vi "Configure Session.vi"(8 "error in":errorcluster, 11 "Plugin in":refnum<class "StreamWriter.lvclass">) -> (0 "error out":errorcluster, 3 "Plugin out":refnum<class "StreamWriter.lvclass">)   [LabVIEW 2024, in "StreamWriter.lvlib" / "StreamWriter.lvclass"]
uses:
  StreamWriter.lvclass
  C:/Program Files/National Instruments/LabVIEW 2024/vi.lib/FlexLogger/SDK/PluginSDK.lvlibp/PEFClasses/SDK/Plugin/Plugin.lvclass
  StreamWriter Parameters.ctl
  StreamWriter.lvclass/StreamWriter.ctl
  StreamWriter Strings.vi
  <vilib>/FlexLogger/SDK/PluginSDK.lvlibp/PEFClasses/SDK/Plugin/ParameterAccess/Read I32.vi
  <vilib>/FlexLogger/SDK/PluginSDK.lvlibp/PEFClasses/SDK/Plugin/Plugin.lvclass
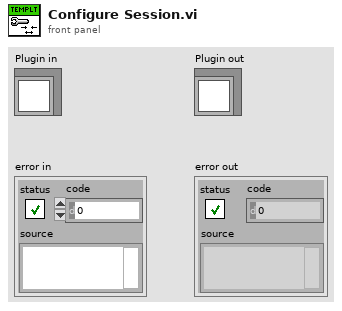
[diagram p1: front panel]
types:
  T1 = typedef "StreamWriter.lvlib/StreamWriter.lvclass/StreamWriter Parameters.ctl" = cluster{"Timeout":i32, "Buffer Size":i32, "Writer Endpoint":refnum<k21>}
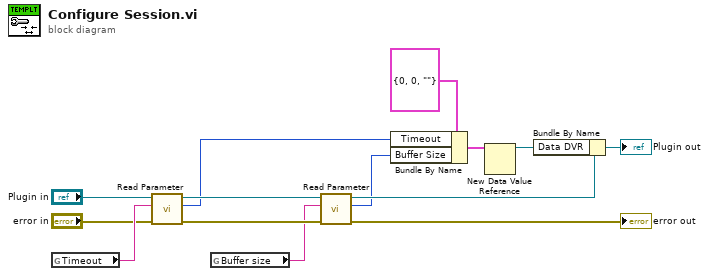
[diagram p0: block diagram]
diagram:
  n1 = global read "StreamWriter Strings.vi" "Timeout"() -> (w5:string)
  n2 = call-poly <vilib>:"Read Parameter.vi"("error in (no error)"="error in", "Name"=w5, "Plugin in"="Plugin in") -> ("error out"=w13:errorcluster, "Value"=w11:i32, "Plugin out"=w14:refnum<class "StreamWriter.lvclass">)  [unwired: 5 in, 1 out]
  n3 = global read "StreamWriter Strings.vi" "Buffer size"() -> (w4:string)
  n4 = call-poly <vilib>:"Read Parameter.vi"("error in (no error)"=w13, "Name"=w4, "Plugin in"=w14) -> ("error out"=→"error out":errorcluster, "Value"=w3:i32, "Plugin out"=w9:refnum<class "StreamWriter.lvclass">)  [unwired: 5 in, 1 out]
  n5 = Bundle By Name(cluster=T1 {"Timeout"=0, "Buffer Size"=0, "Writer Endpoint"=""} ("StreamWriter Parameters"), "Timeout"=w11, "Buffer Size"=w3) -> (w12:T1)
  n6 = New Data Value Reference(data value=w12) -> (data value reference=w8:refnum<data-value>)  [unwired: 1 in, 1 out]
  n7 = Bundle By Name(cluster=w9, "Data DVR"=w8) -> (→"Plugin out":refnum<class "StreamWriter.lvclass">)
